vi "startMission.vi"(8 "error in (no error)":errorcluster, 11 "GenericMission in":refnum<class "GenericMission.lvclass">) -> (0 "error out":errorcluster, 3 "GenericMission out":refnum<class "GenericMission.lvclass">)   [LabVIEW 2011, in "GenericMission.lvclass"]
doc: "Performs a start-up sequence for a mission. This method should always be called once a new mission has begun.\n\nNote: This is a dynamic dispatch method of GenericMission. The correct method will be called based on the run-time class of this object, a child class of GenericMission.\n\nAuthor: Jared Kirschner"
uses:
  GenericMission.lvclass
  2 Globals/2 Message Logger.vi
  Logger/Logger.lvclass
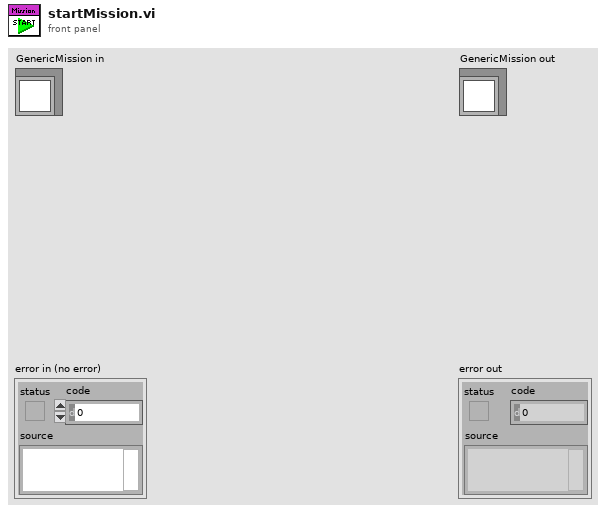
[diagram p1: front panel]
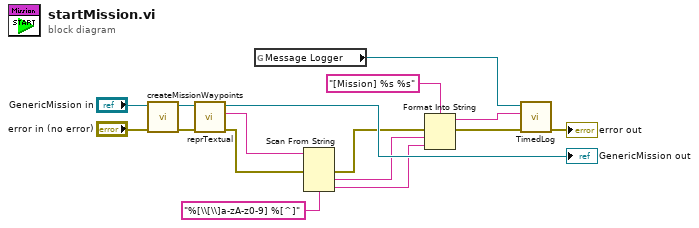
[diagram p0: block diagram]
diagram:
  n1 = call-dynamic "createMissionWaypoints.vi"("error in (no error)"="error in (no error)", "GenericMission in"="GenericMission in") -> ("error out"=w11:errorcluster, "GenericMission out"=w12:refnum<class "GenericMission.lvclass">)  [unwired: 8 in]
  n2 = call-dynamic "reprTextual.vi"("error in (no error)"=w11, "GenericMission in"=w12) -> ("error out"=w4:errorcluster, "Description"=w6:string, "GenericMission out"=→"GenericMission out":refnum<class "GenericMission.lvclass">)  [unwired: 7 in]
  n3 = global read "2 Message Logger.vi" "Message Logger"() -> (w14:refnum<class "Logger.lvclass">)
  n4 = Scan From String(format string="%[\\[\\]a-zA-z0-9] %[^]", input string=w6, error in=w4) -> (error out=w3:errorcluster, output 1=w2:string, output 2=w1:string)  [unwired: 3 in, 2 out]
  n5 = Format Into String(format string="[Mission] %s %s", error in=w3, w2, w1) -> (resulting string=w7:string, error out=w9:errorcluster)  [unwired: 1 in]
  n6 = call "TimedLog.vi"("error in (no error)"=w9, "Message"=w7, "Logger in"=w14) -> ("error out"=→"error out":errorcluster)  [unwired: 6 in, 2 out]
